vi "SS2 Live_Save-Load Settings.vi"(6 "Load(F)/Save (T)":bool, 8 "Error In":errorcluster, 9 "App Name":string, 10 "File Path":path) -> (0 "Error Out":errorcluster, 2 "File Path out":path)   [LabVIEW 2019]
doc: "Use this file to Save or Load AlliGator's settings to an ini file.\nIf the Path input is left unconnected, the defaut ini file is used (overriding the current ini file).\nTo save settings in a user-specified location, either provide a valid path, or connect a \"Not a Path\" constant to the input. A File Dialog window will then open to allow the user to choose a path."
uses:
  SS2 Live_Settings List.ctl
  <vilib>/Utility/sysdir.llb/System Directory Type.ctl
  49d39d47-0c92-4e52-98e4-9eb8d23bbfb7.vi
  <vilib>/Utility/config.llb/NI_LVConfig.lvlib
panel:
  in  "Settings List":T1
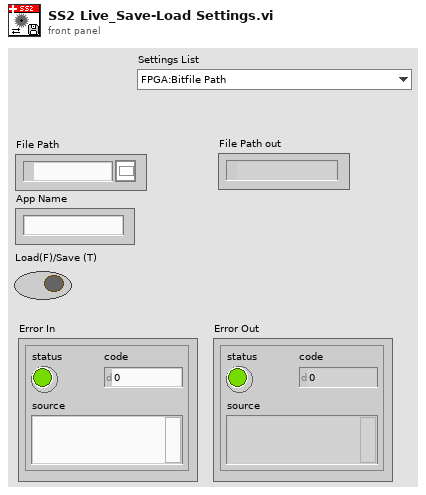
[diagram p1: front panel]
types:
  T1 = typedef "SS2 Live_Settings List.ctl" = enum16{"FPGA:Bitfile Path", "FPGA:Bitfile Version", "Acquisition Parameters:SS2 DAQ Parameters", "Acquisition Parameters:Gate Configuration Array", "Acquisition Parameters:Buffer Size (# Gates)", "File Information:File Information", "File Information:# Datasets in Series", "Image Parameters:Image ROI Information", "Image Parameters:Image Binning Options", "UI Parameters:Histogram Bins Number"}
  T2 = typedef "System Directory Type.ctl" = i32
  T3 = typedef "NI_LVConfig.lvlib/Config Data RefNum.ctl" = refnum<k1>
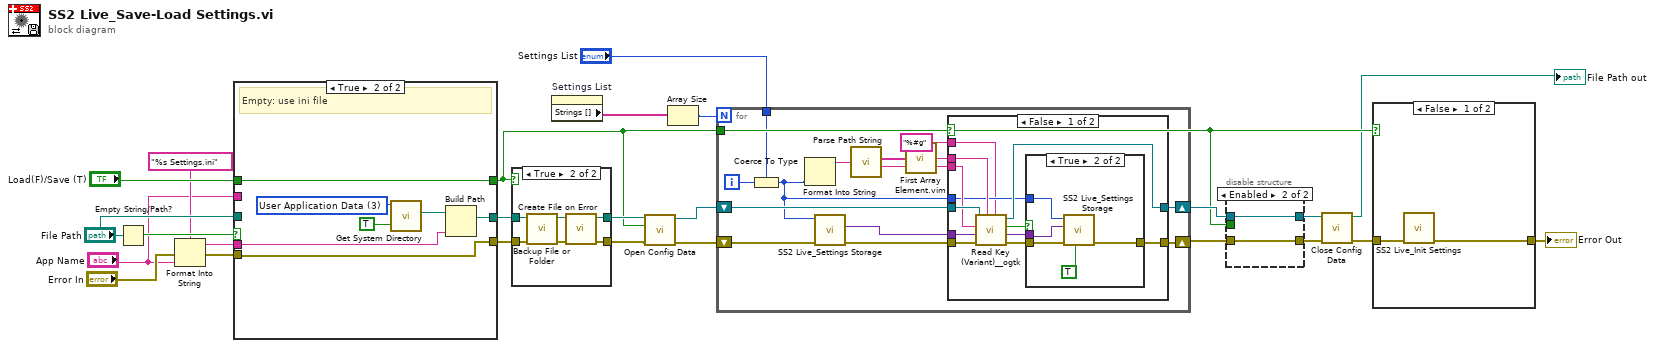
[diagram p0: block diagram]
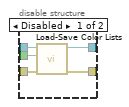
[diagram p2: hidden frame]
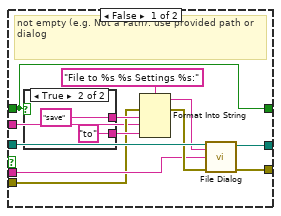
[diagram p3: hidden frame]
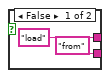
[diagram p4: hidden frame]
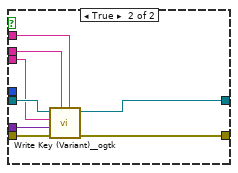
[diagram p7: hidden frame]
diagram:
  n1 = Empty String/Path?(string/path="File Path") -> (empty?=w12:bool)
  n2 = Format Into String(format string="%s Settings.ini" ("name or relative path"), error in="Error In", "App Name") -> (resulting string=w5:string, error out=w3:errorcluster)  [unwired: 1 in]
  n3 = case shown="True" w12 {
    tunnel: [w36 w45] -> w25
    tunnel: [w35 w42] -> w11
    tunnel: "File Path" -> [w37 _]
    tunnel: "Load(F)/Save (T)" -> [w29 w44]
    tunnel: [w29 w44] -> w8
    tunnel: w5 -> [w28 w43]
    tunnel: w3 -> [w27 w42]
    tunnel: "App Name" -> [w26 _]
    frame False {
      # "not empty (e.g. Not a Path): use provided path or dialog"
      n4 = case shown="True" w29 {
        tunnel: ["load" ("input 1") "save" ("input 1")] -> w31
        tunnel: ["from" ("input 2") "to" ("input 2")] -> w30
        frame False {
        }
        frame True {
        }
      }
      n5 = Format Into String(format string="File to %s %s Settings %s:" ("prompt"), error in=w27, w31, w26, w30) -> (resulting string=w33:string, error out=w32:errorcluster)  [unwired: 1 in]
      n6 = call "File Dialog"("start path"=w37, "prompt"=w33, "default name"=w28, "error in"=w32) -> ("selected path"=w36:path, "error out"=w35:errorcluster)  [unwired: 8 in, 2 out]
    }
    frame True {
      w46 = T2 3 items=["User Home"=0, "User Desktop"=1, "User Documents"=2, "User Application Data"=3, "User Preferences"=4, "User Temporary"=5, "Public Documents"=6, "Public Application Data"=7, "Public Preferences"=8, "Public Cache"=13, "System Core Libraries"=9, "System Installed Libraries"=10, "Application Files"=11, "Boot Volume Root"=12] ("system directory type")
      # "Empty: use ini file"
      n7 = call <vilib>:"Get System Directory.vi"("create directory if not found? (F)"=TRUE, "system directory type"=w46) -> ("system directory"=w47:path)  [unwired: 9 in]
      n8 = Build Path(base path=w47, name or relative path=w43) -> (appended path=w45:path)
    }
  }
  n9 = case shown="True" w8 {
    tunnel: w25 -> [w50 w56]
    tunnel: w11 -> [w49 w55]
    tunnel: [w50 w52] -> w24
    tunnel: [w49 w51] -> w23
    frame False {
    }
    frame True {
      n10 = call "Backup File or Folder.vi"("error in (no error)"=w55, "File/Directory Path"=w56) -> ("error out"=w53:errorcluster, "File/Directory Path (dup)"=w54:path)  [unwired: 8 in]
      n11 = call "Create File on Error.vi"("error in (no error)"=w53, "File Path"=w54) -> ("error out"=w51:errorcluster, "File Path (dup)"=w52:path)  [unwired: 8 in]
    }
  }
  n12 = property on="Settings List" class="Enum (strict)"() -> ("Strings []"=w19:string[])  [unwired: 2 in, 2 out]
  n13 = call <vilib>:"Open Config Data.vi"("error in (no error)"=w23, "create file if necessary (T)"=w8, "configuration file path"=w24) -> ("error out"=w22:errorcluster, "refnum"=w21:T3)  [unwired: 6 in, 1 out]
  n14 = Array Size(array=w19) -> (size(s)=w18:i32)
  n15 = for {
    N: w18 -> [_]
    shift-right: [w66] -> w15
    shift-left: w22 -> [w59]
    shift-right: [w67] -> w16
    shift-left: w21 -> [w68]
    tunnel: "Settings List" -> [w70]
    tunnel: w8 -> [w69]
    i -> [w71]
    n16 = Coerce To Type(0:w71, 1:w70) -> (2:w60:T1)
    n17 = Format Into String(w60) -> (resulting string=w65:string)  [unwired: 3 in, 1 out]
    n18 = call "SS2 Live_Settings Storage.vi"("Error In"=w59, "Settings List"=w60) -> ("Error Out"=w58:errorcluster, "Variant Data out"=w57:variant)  [unwired: 8 in]
    n19 = call "Parse Path String.vi"("Path in"=w65) -> ("Folder Hierarchy"=w63:string[], "File/Folder"=w64:string)  [unwired: 4 in]
    n20 = call "First Array Element.vim"("Array"=w63) -> ("First Element"=w62:string)  [unwired: 8 in]
    n21 = case shown="False" w69 {
      tunnel: w68 -> [w83 w97]
      tunnel: [w80 w96] -> w67
      tunnel: w57 -> [w82 w93]
      tunnel: w58 -> [w81 w95]
      tunnel: [w76 w94] -> w66
      tunnel: w64 -> [w79 w92]
      tunnel: w62 -> [w78 w91]
      tunnel: w60 -> [w75 _]
      tunnel: "%#g" ("float number format") -> [w72 w90]
      frame False {
        n22 = call <userlib>:"Read Key (Variant)__ogtk.vi"("format string (%;%f)"=w72, "section"=w78, "error in (no error)"=w81, "type"=w82, "key (optional)"=w79, "refnum"=w83) -> ("error out"=w77:errorcluster, "key-value"=w74:variant, "found?"=w73:bool, "refnum out"=w80:T3)  [unwired: 2 in]
        n23 = case shown="True" w73 {
          tunnel: w77 -> [w84 w89]
          tunnel: [w84 w87] -> w76
          tunnel: w75 -> [_ w85]
          tunnel: w74 -> [_ w86]
          frame False {
          }
          frame True {
            n24 = call "SS2 Live_Settings Storage.vi"("Set/Get(F)"=TRUE ("Get (F)/Set"), "Error In"=w89, "Variant Data in"=w86, "Settings List"=w85) -> ("Error Out"=w87:errorcluster)  [unwired: 6 in, 1 out]
          }
        }
      }
      frame True {
        n25 = call <userlib>:"Write Key (Variant)__ogtk.vi"("float number format"=w90, "section"=w91, "error in (no error)"=w95, "key-value"=w93, "key (optional)"=w92, "refnum"=w97) -> ("error out"=w94:errorcluster, "refnum out"=w96:T3)  [unwired: 4 in]
      }
    }
  }
  n26 = disable-structure shown="Enabled" {
    disable-tunnel: w16 -> [w102 w104]
    disable-tunnel: w15 -> [w101 w103]
    disable-tunnel: [w100 w104] -> w14
    disable-tunnel: [w99 w103] -> w13
    disable-tunnel: w8 -> [w98 _]
    frame Disabled {
      n27 = call "Load-Save Color Lists.vi"("error in (no error)"=w101, "Load (F)/Save"=w98, "ini File Refnum in"=w102) -> ("error out"=w99:errorcluster, "ini File Refnum out"=w100:T3)  [unwired: 7 in]
    }
    frame Enabled {
    }
  }
  n28 = call <vilib>:"Close Config Data.vi"("error in (no error)"=w13, "refnum"=w14) -> ("error out"=w20:errorcluster, "file path"=→"File Path out":path)  [unwired: 8 in]
  n29 = case shown="False" w8 {
    tunnel: w20 -> [w106 w107]
    tunnel: [w105 w107] -> w17
    frame False {
      n30 = call "SS2 Live_Init Settings.vi"("error in (no error)"=w106) -> ("error out"=w105:errorcluster)  [unwired: 10 in]
    }
    frame True {
    }
  }
  "Error Out" <- w17
